vi "BatteryCyclingGlobalDAQ3.vi"() -> ()   [LabVIEW 2020]
uses:
  <instrlib>/NH Research Regenerative Test Series/Public/Configure/Output Safety.ctl
  Readings.vi
  <instrlib>/NH Research Regenerative Test Series/Public/Data/Read (Ave Current).vi
  <instrlib>/NH Research Regenerative Test Series/Public/Data/Low Level/Fetch (Ave Voltage).vi
  <instrlib>/NH Research Regenerative Test Series/Public/Data/Low Level/Fetch (Ave True Power).vi
  <instrlib>/NH Research Regenerative Test Series/NH Research Regenerative Test Series.lvlib
panel:
  in  "Starting Cycle":i32
  out "Battemp 2":dbl
  out "AmbientTemp":dbl
  out "Tab Control 2":T1(tab)
  out "Selected Output Safety 2":T2
  in  "Custom Output Safety 2":T2
  out "Discharge Rest Voltage":dbl(graph)
  out "Charge Rest Voltage":dbl(graph)
  out "Ave Current (A)":dbl
  out "Ave Voltage (V)":dbl
  out "Ave True Power (W)":dbl
  out "Battemp":dbl
  out "HoopStrain":dbl
  in  "Tab Control":T1(tab)
  out "Selected Output Safety":T2
  in  "Custom Output Safety":T2
  in  "Output Safety\nSelection":bool caption="Output Safety"
  in  "Non Default Folder Path":path
  in  "Cycling Test Folder Name":string
  in  "NHR VISA Name":refnum<visa-resource-name>
  out "Error Out":string
  out "Previous Discharge Data File":path caption="Filename Out"
  out "Previous Charge Data File":path caption="Filename Out"
  out "D Wait Status Byte Register":T3
  out "Discharge Status Byte Register":T3
  out "C Wait Status Byte Register":T3
  out "Charge Status Byte Register":T3
  in  "Cycle Stop":bool
  out "Cycle Index":i32
  in  "Number of Cycles":i32
  out "Discharge Rest":bool
  in  "Wait Time":u32
  out "Discharge Rest Voltage":dbl
  out "Elaspsed Time":u32 caption="Elapsed Time (s)"
  out "Charge Rest":bool
  in  "Wait Time":u32
  out "Charge Rest Voltage":dbl
  out "Elapsed Time":u32 caption="Elapsed Time (s)"
  out "Discharging":bool
  in  "Discharge Stop":bool
  in  "Discharge Current":dbl
  in  "Voltage Cutoff":dbl
  out "Charging":bool
  in  "Charge Stop":bool
  in  "Current Cutoff":dbl
  in  "Charge Current":dbl format="%#.6g"
  in  "Charge Voltage":dbl format="%#.6g"
  in  "Logical Instrument Number":u32=1
  # "Test Name & Device Info"
  # "Error Indication"
  # "Rest Voltage Charts"
  # "Readings"
  # "Output Safety Configuration"
  # "Cycle & Charge Profile Settings"
  # "Cycle\nInfo"
  # "Post Discharge\nRest"
  # "Post Charge\nRest"
  # "Discharging"
  # "Charging"
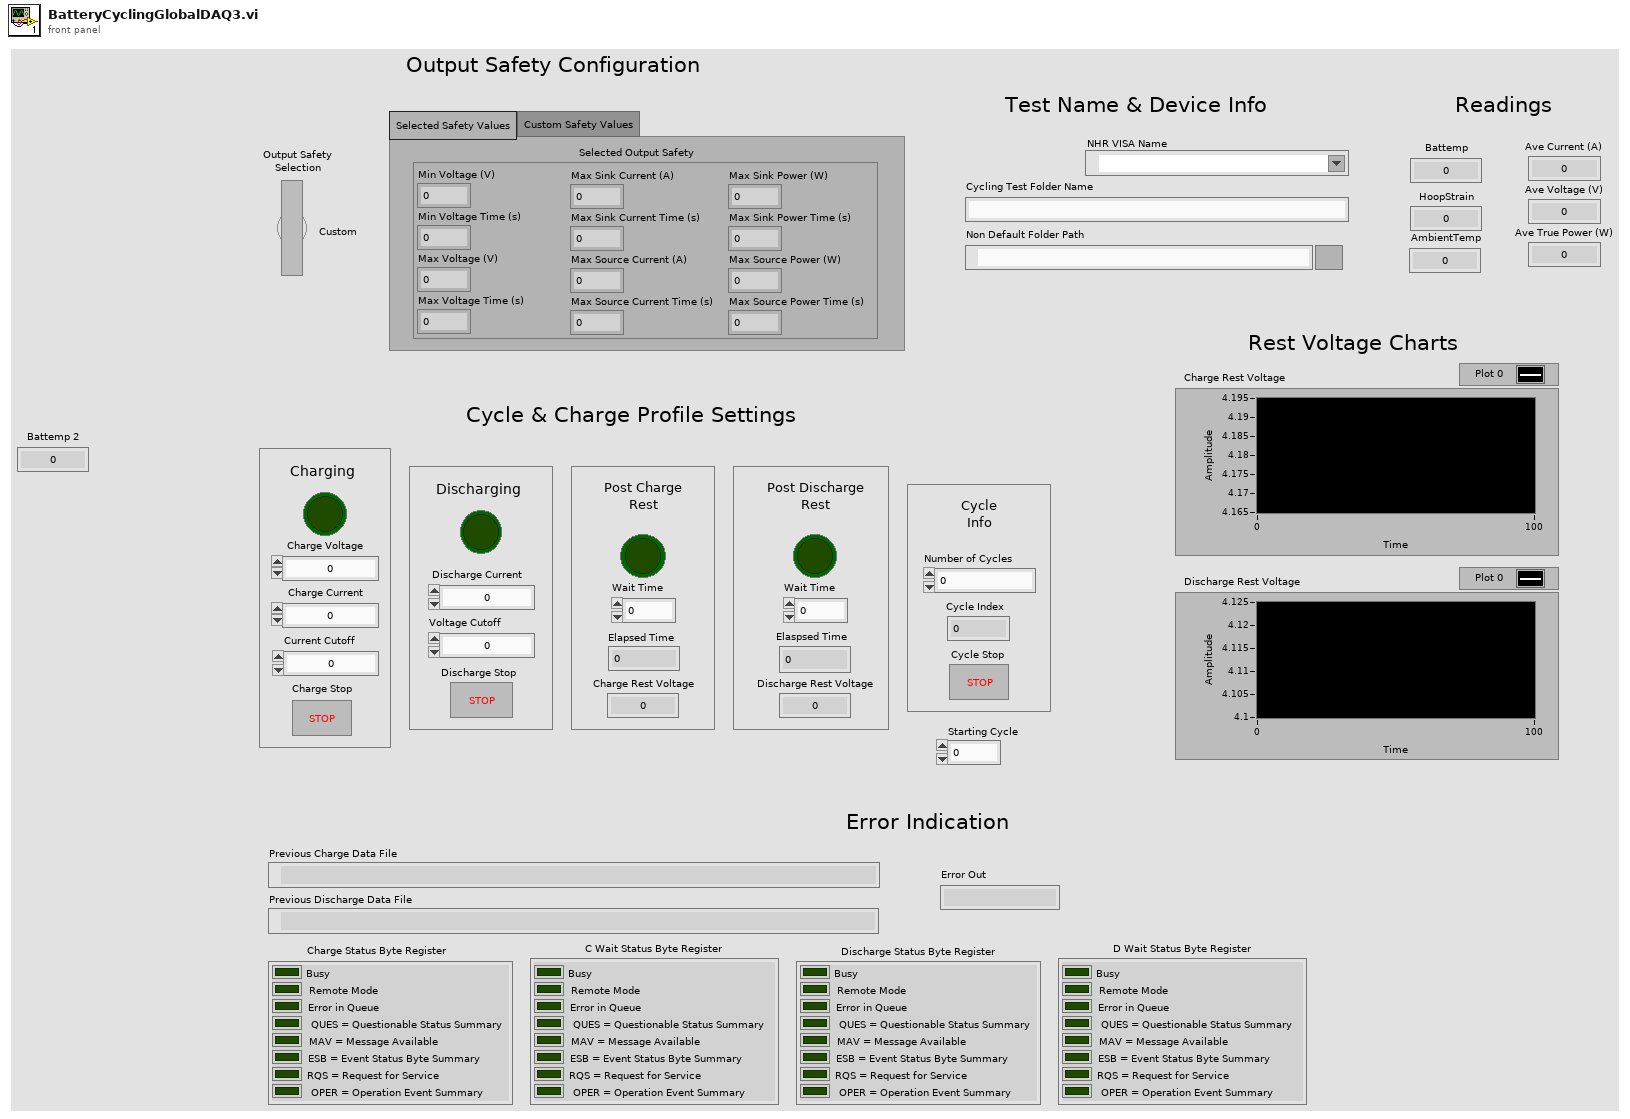
[diagram p1: front panel]
types:
  T1 = enum32{"Selected Safety Values", "Custom Safety Values"}
  T2 = typedef "NH Research Regenerative Test Series.lvlib/Output Safety.ctl" = cluster{"Min Voltage (V)":dbl, "Min Voltage Time (s)":dbl, "Max Voltage (V)":dbl, "Max Voltage Time (s)":dbl, "Max Sink Current (A)":dbl, "Max Sink Current Time (s)":dbl, "Max Source Current (A)":dbl, "Max Source Current Time (s)":dbl, "Max Sink Power (W)":dbl, "Max Sink Power Time (s)":dbl, "Max Source Power (W)":dbl, "Max Source Power Time (s)":dbl}
  T3 = cluster{"Busy":bool, "Remote Mode":bool, "Error in Queue":bool, "QUES = Questionable Status Summary":bool, "MAV = Message Available":bool, "ESB = Event Status Byte Summary":bool, "RQS = Request for Service":bool, "OPER = Operation Event Summary":bool}
  T4 = cluster{"Min Voltage (V)":dbl, "Min Voltage Time (s)":dbl, "Max Voltage (V)":dbl, "Max Voltage Time (s)":dbl, "Max Sink Current (A)":dbl, "Max Sink Current Time (s)":dbl, "Max Source Current (A)":dbl, "Max Source Current Time (s)":dbl, "Max Sink Power (W)":dbl, "Max Sink Power Time (s)":dbl, "Max Source Power (W)":dbl, "Max Source Power Time (s)":dbl}
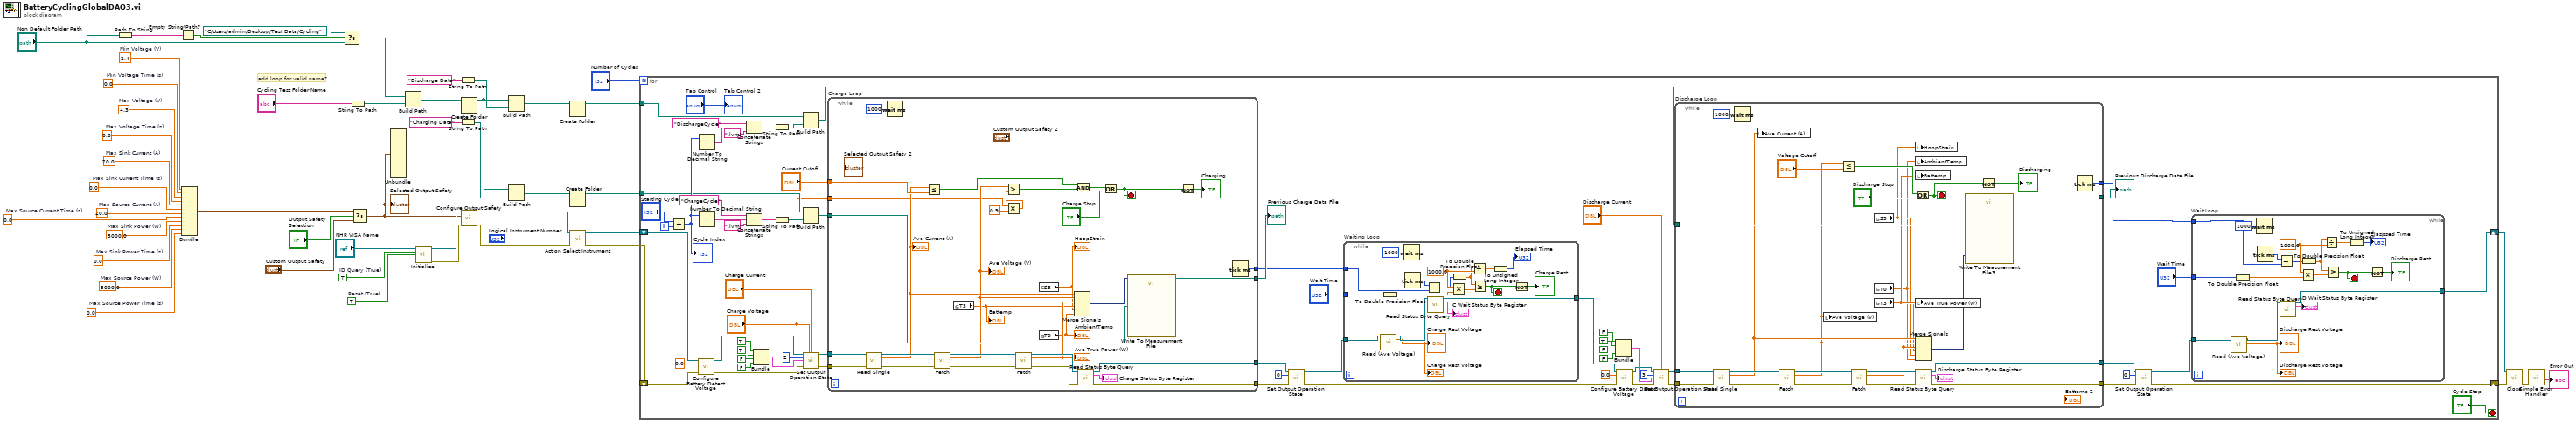
[diagram p0: block diagram]
diagram:
  w23 = 5000.0  # Max Source Power (W)
  w24 = 0.0  # Max Sink Power Time (s)
  w25 = 5000.0  # Max Sink Power (W)
  w26 = 0.0  # Max Source Current Time (s)
  w27 = 20.0  # Max Source Current (A)
  w29 = 20.0  # Max Sink Current (A)
  w28 = 0.0  # Max Sink Current Time (s)
  w30 = 0.0  # Max Voltage Time (s)
  w31 = 4.3  # Max Voltage (V)
  w32 = 2.4  # Min Voltage (V)
  w22 = 0.0  # Max Source Power Time (s)
  w33 = 0.0  # Min Voltage Time (s)
  w47 = TRUE  # ID Query (True)
  w46 = TRUE  # Reset (True)
  # "add loop for valid name?"
  n1 = Path To String(path="Non Default Folder Path") -> (string=w7:string)
  n2 = Empty String/Path?(string/path=w7) -> (empty?=w6:bool)
  n3 = Bundle("Min Voltage (V)"=w32, "Min Voltage Time (s)"=w33, "Max Voltage (V)"=w31, "Max Voltage Time (s)"=w30, "Max Sink Current (A)"=w29, "Max Sink Current Time (s)"=w28, "Max Source Current (A)"=w27, "Max Source Current Time (s)"=w26, "Max Sink Power (W)"=w25, "Max Sink Power Time (s)"=w24, "Max Source Power (W)"=w23, "Max Source Power Time (s)"=w22) -> (w20:T4)  [unwired: 1 in]
  n4 = Select(t=path "C:/Users/admin/Desktop/Test Data/Cycling", s=w6, f="Non Default Folder Path") -> (s? t:f=w10:path)
  n5 = String To Path(string="Cycling Test Folder Name") -> (path=w12:path)
  n6 = Select(t=w20, s="Output Safety\nSelection", f="Custom Output Safety") -> (s? t:f=w21:T2)
  "Selected Output Safety" <- w21
  n7 = Unbundle(w21) -> ()  [unwired: 12 out]
  n8 = Build Path(base path=w10, name or relative path=w12) -> (appended path=w9:path)
  n9 = call <instrlib>:"Initialize.vi"("VISA resource name"="NHR VISA Name", "ID Query (True)"=w47, "Reset (True)"=w46) -> ("VISA resource name out"=w45:refnum<visa-resource-name>, "error out"=w44:errorcluster)  [unwired: 11 in]
  n10 = String To Path(string="Discharge Data") -> (path=w15:path)
  n11 = String To Path(string="Charging Data") -> (path=w13:path)
  n12 = Create Folder(path (use dialog)=w9) -> (created path=w17:path)  [unwired: 2 in, 2 out]
  n13 = call <instrlib>:"Configure Output Safety.vi"("VISA resource name"=w45, "Output Safety"=w21, "error in (no error)"=w44) -> ("VISA resource name out"=w42:refnum<visa-resource-name>, "error out"=w41:errorcluster)  [unwired: 11 in]
  n14 = Build Path(base path=w17, name or relative path=w15) -> (appended path=w16:path)
  n15 = Build Path(base path=w17, name or relative path=w13) -> (appended path=w14:path)
  n16 = Create Folder(path (use dialog)=w16) -> (created path=w2:path)  [unwired: 2 in, 2 out]
  n17 = Create Folder(path (use dialog)=w14) -> (created path=w1:path)  [unwired: 2 in, 2 out]
  n18 = call <vilib>:"Action Select Instrument.vi"("VISA resource name"=w42, "Logical Instrument Number"="Logical Instrument Number", "error in (no error)"=w41) -> ("VISA resource name out"=w38:refnum<visa-resource-name>, "error out"=w37:errorcluster)  [unwired: 11 in]
  n19 = for {
    N: "Number of Cycles" -> [_]
    shift-right: [w73] -> w36
    shift-left: w38 -> [w81]
    shift-right: [w76] -> w35
    shift-left: w37 -> [w79]
    tunnel: w2 -> [w53]
    tunnel: w1 -> [w52]
    i -> [w77]
    stop <- "Cycle Stop" stop-if-true
    n20 = Add(x="Starting Cycle", y=w77) -> (x+y=w58:i32)
    "Cycle Index" <- w58
    n21 = call <instrlib>:"Configure Battery Detect Voltage.vi"("VISA resource name"=w81, "Battery Detect Voltage (0V)"=0.0, "error in (no error)"=w79) -> ("VISA resource name out"=w80:refnum<visa-resource-name>, "error out"=w78:errorcluster)  [unwired: 11 in]
    n22 = Number To Decimal String(number=w58) -> (decimal integer string=w62:string)  [unwired: 1 in]
    n23 = Number To Decimal String(number=w58) -> (decimal integer string=w67:string)  [unwired: 1 in]
    n24 = Concatenate Strings("DischargeCycle", w62, ".lvm") -> (w60:string)
    n25 = Concatenate Strings("ChargeCycle", w67, ".lvm") -> (w64:string)
    n26 = Bundle(TRUE, TRUE, FALSE, FALSE) -> (w82:cluster{bool, bool, bool, bool})  [unwired: 1 in]
    n27 = String To Path(string=w60) -> (path=w57:path)
    n28 = String To Path(string=w64) -> (path=w65:path)
    n29 = Build Path(base path=w53, name or relative path=w57) -> (appended path=w69:path)
    n30 = Build Path(base path=w52, name or relative path=w65) -> (appended path=w54:path)
    n31 = call <instrlib>:"Set Output Operation State.vi"("VISA resource name"=w80, "Voltage Setpoint (0 V)"="Charge Voltage", "Current Setpoint (0 A)"="Charge Current", "Mode (0: Off)"=2, "Enable"=w82, "error in (no error)"=w78) -> ("VISA resource name out"=w89:refnum<visa-resource-name>, "error out"=w88:errorcluster)  [unwired: 8 in]
    n32 = while "Charge Loop" {
      tunnel: w89 -> [w202]
      tunnel: w88 -> [w201]
      tunnel: [w199] -> w96
      tunnel: [w198] -> w95
      tunnel: "Current Cutoff" -> [w194]
      tunnel: w54 -> [w188]
      tunnel: [w195] -> w113
      tunnel: [w189] -> w71
      tunnel: "Charge Voltage" -> [w178]
      stop <- w185 stop-if-true
      n33 = call-poly <instrlib>:"Read Single.vi"("VISA resource name"=w202, "error in (no error)"=w201) -> ("VISA resource name out"=w207:refnum<visa-resource-name>, "Ave Current (A)"=w193:dbl, "error out"=w208:errorcluster)  [unwired: 11 in]
      "Ave Current (A)" <- w193
      n34 = Wait (ms)(milliseconds to wait=1000) -> ()  [unwired: 1 out]
      n35 = Less Or Equal?(x=w193, y=w194) -> (x <= y?=w191:bool)
      n36 = call-poly <instrlib>:"Fetch.vi"("VISA resource name"=w207, "error in (no error)"=w208) -> ("VISA resource name out"=w206:refnum<visa-resource-name>, "Ave Voltage (V)"=w183:dbl, "error out"=w205:errorcluster)  [unwired: 11 in]
      "Ave Voltage (V)" <- w183
      n37 = global read "Readings.vi" "T3"() -> (w182:dbl)
      "Battemp" <- w182
      n38 = Multiply(x=w178, y=0.9) -> (x*y=w177:dbl)
      n39 = Greater?(x=w183, y=w177) -> (0:w190:bool)
      n40 = call-poly <instrlib>:"Fetch.vi"("VISA resource name"=w206, "error in (no error)"=w205) -> ("VISA resource name out"=w204:refnum<visa-resource-name>, "Ave True Power (W)"=w197:dbl, "error out"=w203:errorcluster)  [unwired: 11 in]
      "Ave True Power (W)" <- w197
      n41 = global read "Readings.vi" "S3"() -> (w181:dbl)
      "HoopStrain" <- w181
      n42 = global read "Readings.vi" "T0"() -> (w180:dbl)
      "AmbientTemp" <- w180
      n43 = Merge Signals "Merge Signals"(w193, w183, w197, w182, w181, w180) -> (w196:dynamicdata)
      n44 = And(x=w191, y=w190) -> (x .and. y?=w187:bool)
      n45 = call <instrlib>:"Read Status Byte Query.vi"("VISA resource name"=w204, "error in (no error)"=w203) -> ("VISA resource name out"=w199:refnum<visa-resource-name>, "Status Byte Register"=→"Charge Status Byte Register":T3, "error out"=w198:errorcluster)  [unwired: 11 in]
      n46 = Or(x=w187, y="Charge Stop") -> (x .or. y?=w185:bool)
      n47 = call "Write To Measurement File"("Signals"=w196, "Filename"=w188) -> ("Filename Out"=w195:path)  [unwired: 15 in, 2 out]
      n48 = Not(x=w185) -> (.not. x?=→"Charging":bool)
      n49 = Tick Count (ms)() -> (millisecond timer value=w189:u32)
    }
    "Previous Charge Data File" <- w113
    n50 = call <instrlib>:"Set Output Operation State.vi"("VISA resource name"=w96, "Mode (0: Off)"=0, "error in (no error)"=w95) -> ("VISA resource name out"=w92:refnum<visa-resource-name>, "error out"=w94:errorcluster)  [unwired: 11 in]
    n51 = while "Waiting Loop" {
      tunnel: [w175] -> w98
      tunnel: "Wait Time" -> [w163]
      tunnel: w71 -> [w172]
      tunnel: w92 -> [w159]
      stop <- w168 stop-if-true
      w173 = 1000.0
      n52 = call <instrlib>:"Read (Ave Voltage).vi"("VISA resource name"=w159) -> ("VISA resource name out"=w161:refnum<visa-resource-name>, "Ave Voltage (V)"=→"Charge Rest Voltage" →"Charge Rest Voltage":dbl)  [unwired: 12 in, 1 out]
      n53 = To Double Precision Float(number=w163) -> (double precision float=w162:dbl)
      n54 = Wait (ms)(milliseconds to wait=1000) -> ()  [unwired: 1 out]
      n55 = Tick Count (ms)() -> (millisecond timer value=w171:u32)
      n56 = Subtract(x=w171, y=w172) -> (x-y=w165:u32)
      n57 = call <instrlib>:"Read Status Byte Query.vi"("VISA resource name"=w161) -> ("VISA resource name out"=w175:refnum<visa-resource-name>, "Status Byte Register"=→"C Wait Status Byte Register":T3)  [unwired: 12 in, 1 out]
      n58 = Multiply(x=w173, y=w162) -> (x*y=w174:dbl)
      n59 = To Double Precision Float(number=w165) -> (double precision float=w164:dbl)
      n60 = Divide(x=w164, y=w173) -> (x/y=w167:dbl)
      n61 = Greater Or Equal?(x=w164, y=w174) -> (x >= y?=w168:bool)
      n62 = To Unsigned Long Integer(number=w167) -> (unsigned 32bit integer=→"Elapsed Time":u32)
      n63 = Not(x=w168) -> (.not. x?=→"Charge Rest":bool)
    }
    n64 = Bundle(FALSE, TRUE, FALSE, FALSE) -> (w104:cluster{bool, bool, bool, bool})  [unwired: 1 in]
    n65 = call <instrlib>:"Configure Battery Detect Voltage.vi"("VISA resource name"=w98, "Battery Detect Voltage (0V)"=0.0, "error in (no error)"=w94) -> ("VISA resource name out"=w97:refnum<visa-resource-name>, "error out"=w99:errorcluster)  [unwired: 11 in]
    n66 = call <instrlib>:"Set Output Operation State.vi"("VISA resource name"=w97, "Current Setpoint (0 A)"="Discharge Current", "Mode (0: Off)"=3, "Enable"=w104, "error in (no error)"=w99) -> ("VISA resource name out"=w109:refnum<visa-resource-name>, "error out"=w110:errorcluster)  [unwired: 9 in]
    n67 = while "Discharge Loop" {
      tunnel: w109 -> [w152]
      tunnel: w110 -> [w151]
      tunnel: [w149] -> w102
      tunnel: [w148] -> w101
      tunnel: w69 -> [w147]
      tunnel: [w145] -> w75
      tunnel: [w143] -> w70
      stop <- w138 stop-if-true
      n68 = call-poly <instrlib>:"Read Single.vi"("VISA resource name"=w152, "error in (no error)"=w151) -> ("VISA resource name out"=w157:refnum<visa-resource-name>, "Ave Current (A)"=w137:dbl, "error out"=w158:errorcluster)  [unwired: 11 in]
      n69 = Wait (ms)(milliseconds to wait=1000) -> ()  [unwired: 1 out]
      n70 = local write "Ave Current (A)"(w137) -> ()
      n71 = call-poly <instrlib>:"Fetch.vi"("VISA resource name"=w157, "error in (no error)"=w158) -> ("VISA resource name out"=w156:refnum<visa-resource-name>, "Ave Voltage (V)"=w136:dbl, "error out"=w155:errorcluster)  [unwired: 11 in]
      n72 = local write "Ave Voltage (V)"(w136) -> ()
      n73 = Less Or Equal?(x=w136, y="Voltage Cutoff") -> (x <= y?=w141:bool)
      n74 = call-poly <instrlib>:"Fetch.vi"("VISA resource name"=w156, "error in (no error)"=w155) -> ("VISA resource name out"=w154:refnum<visa-resource-name>, "Ave True Power (W)"=w135:dbl, "error out"=w153:errorcluster)  [unwired: 11 in]
      n75 = global read "Readings.vi" "S3"() -> (w133:dbl)
      n76 = global read "Readings.vi" "T0"() -> (w132:dbl)
      n77 = global read "Readings.vi" "T3"() -> (w134:dbl)
      n78 = Or(x=w141, y="Discharge Stop") -> (x .or. y?=w138:bool)
      n79 = local write "HoopStrain"(w133) -> ()
      n80 = local write "AmbientTemp"(w132) -> ()
      n81 = local write "Battemp"(w134) -> ()
      n82 = local write "Ave True Power (W)"(w135) -> ()
      n83 = Merge Signals "Merge Signals"(w137, w136, w135, w134, w133, w132) -> (w146:dynamicdata)
      n84 = call <instrlib>:"Read Status Byte Query.vi"("VISA resource name"=w154, "error in (no error)"=w153) -> ("VISA resource name out"=w149:refnum<visa-resource-name>, "Status Byte Register"=→"Discharge Status Byte Register":T3, "error out"=w148:errorcluster)  [unwired: 11 in]
      n85 = call "Write To Measurement File3"("Signals"=w146, "Filename"=w147) -> ("Filename Out"=w145:path)  [unwired: 15 in, 2 out]
      n86 = Not(x=w138) -> (.not. x?=→"Discharging":bool)
      n87 = Tick Count (ms)() -> (millisecond timer value=w143:u32)
    }
    "Previous Discharge Data File" <- w75
    n88 = call <instrlib>:"Set Output Operation State.vi"("VISA resource name"=w102, "Mode (0: Off)"=0, "error in (no error)"=w101) -> ("VISA resource name out"=w74:refnum<visa-resource-name>, "error out"=w76:errorcluster)  [unwired: 11 in]
    n89 = while "Wait Loop" {
      tunnel: [w130] -> w73
      tunnel: "Wait Time" -> [w119]
      tunnel: w70 -> [w127]
      tunnel: w74 -> [w114]
      stop <- w122 stop-if-true
      w128 = 1000.0
      n90 = call <instrlib>:"Read (Ave Voltage).vi"("VISA resource name"=w114) -> ("VISA resource name out"=w116:refnum<visa-resource-name>, "Ave Voltage (V)"=→"Discharge Rest Voltage" →"Discharge Rest Voltage":dbl)  [unwired: 12 in, 1 out]
      n91 = To Double Precision Float(number=w119) -> (double precision float=w118:dbl)
      n92 = Wait (ms)(milliseconds to wait=u32 1000) -> ()  [unwired: 1 out]
      n93 = Tick Count (ms)() -> (millisecond timer value=w126:u32)
      n94 = Subtract(x=w126, y=w127) -> (x-y=w125:u32)
      n95 = call <instrlib>:"Read Status Byte Query.vi"("VISA resource name"=w116) -> ("VISA resource name out"=w130:refnum<visa-resource-name>, "Status Byte Register"=→"D Wait Status Byte Register":T3)  [unwired: 12 in, 1 out]
      n96 = Multiply(x=w128, y=w118) -> (x*y=w129:dbl)
      n97 = To Double Precision Float(number=w125) -> (double precision float=w117:dbl)
      n98 = Divide(x=w117, y=w128) -> (x/y=w121:dbl)
      n99 = Greater Or Equal?(x=w117, y=w129) -> (x >= y?=w122:bool)
      n100 = To Unsigned Long Integer(number=w121) -> (unsigned 32bit integer=→"Elaspsed Time":u32)
      n101 = Not(x=w122) -> (.not. x?=→"Discharge Rest":bool)
    }
    "Tab Control 2" <- "Tab Control"
  }
  n102 = call <instrlib>:"Close.vi"("VISA resource name"=w36, "error in (no error)"=w35) -> ("error out"=w40:errorcluster)  [unwired: 13 in]
  n103 = call <vilib>:"Simple Error Handler.vi"("error in (no error)"=w40) -> ("source out"=→"Error Out":string)  [unwired: 4 in, 4 out]
